vi "4-2 matrice NxM - matrice max - matrice 100x.vi"(0 "colonna\nsize":i32=4, 1 "riga\nsize":i32=3) -> (2 "Array moltiplicazione":dbl[](array[numeric]) format="%#_3g", 3 "Array massimi":dbl[](array[numeric]) format="%#_3g", 4 "Array":dbl[][](array[numeric]) format="%#.2g")   [LabVIEW 2012]
panel:
  out "Waveform Graph":cluster{dbl, dbl, dbl[][]}(graph)
  out "c(i)":dbl[](array[numeric]) format="%#_3g"
  out "b(i)":dbl[](array[numeric]) format="%#_3g"
  out "a(i)":dbl[](array[numeric]) format="%#_3g"
  # "Realizzare, mediante un generatore di numeri casuali,\n una matrice 3xN [a(i), b(i), c(i) con i che varia  da 0 a N-1] con N impostabile da pannello .\n\n Utilizzando la matrice generata dal SubVi precedente, generare due vettori\n  A(i) e B(i)  [0 <= i <= N-1] dove A(i) = Max [a(i),b(i),c(i)]  e B(i) = 100*[b(i) + c(N-1-i)]\n\nVisualizzare in un grafico i vettori a(i), b(i) e A(i)"
  # "DOMANDE: \n- nel ciclo for per la creazione di A(i), con l'indicizzazione abilitata in ingresso, \nil programma confronta automaticamente la prima, poi la seconda e infine la terza\nriga del vettore in ingresso, se invece collego l'indice di Array Subset all'indice del \nciclo, il confronto parte la prima volta dall'elemento 0-0, poi dall'elemento 1-1 e poi dal\n2-2 (che non c' quindi viene passato in uscita 0). Perch? Cosa devo cambiare perch \nfunzioni se l'indicizzazione non  abilitata?\n- nella creazione di B(i), ogni tanto la somma delle componenti non  esatta ( inferiore di 1 unit),\nperch? Il fatto che se rappresento le componenti di B(i) come decimali ottengo cifre sgnificative\ndopo la virgola  dovuto solo al fatto che i numeri random sono generati con molte cifre?"
  # "RISPOSTE:\n- per ottenere lo stesso risultato con l'indicizzazione non abilitata devo fare \"add dimension\" su \"array subset\",\ncollegare l'indice i del ciclo al primo indice di array subset e lasciare scollegato il secondo. Se faccio come nel\ntesto della domanda vengono confrontati gli elementi di uno stesso vettore.\n-  dovuto al fatto che i numeri random sono generati con molte cifre decimali, se la parte decimale supera 5\nil risultato viene arrotondato all'intero successivo."
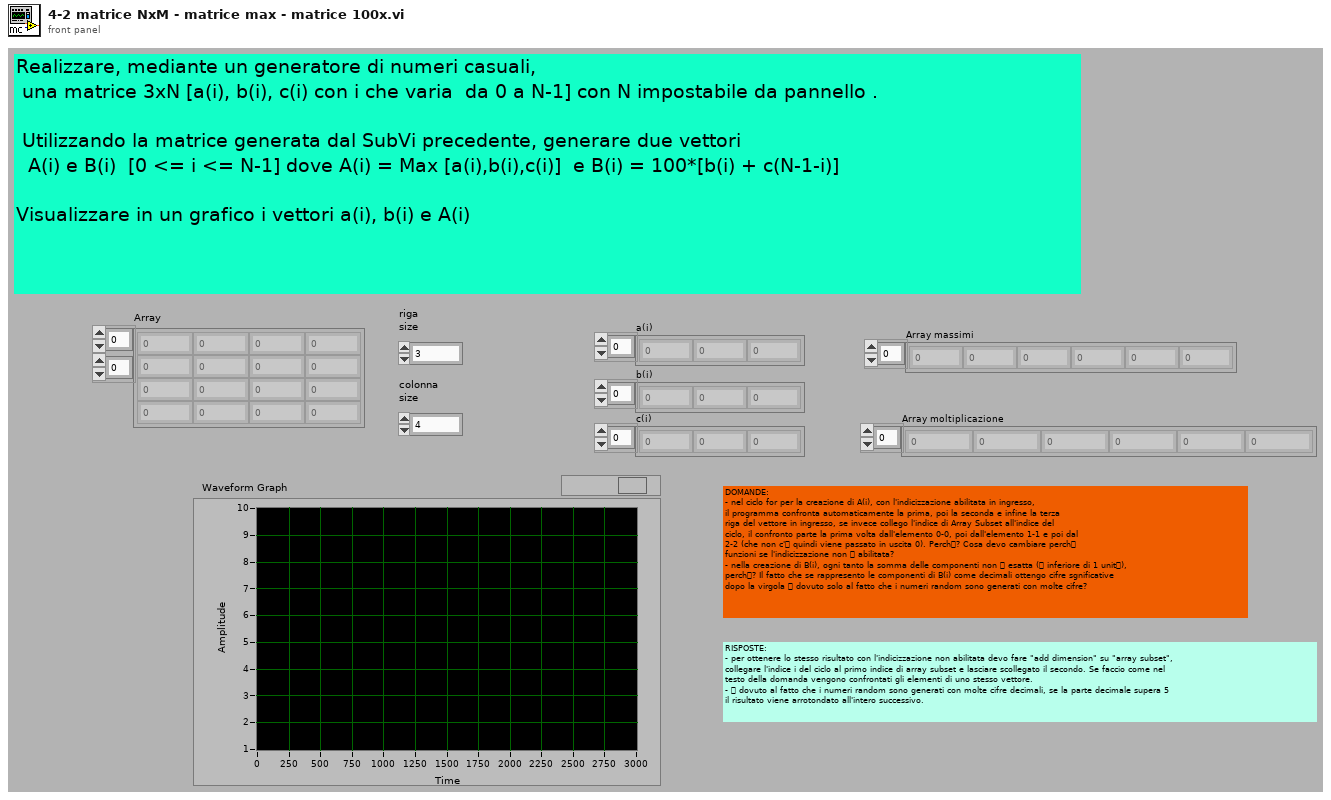
[diagram p1: front panel]
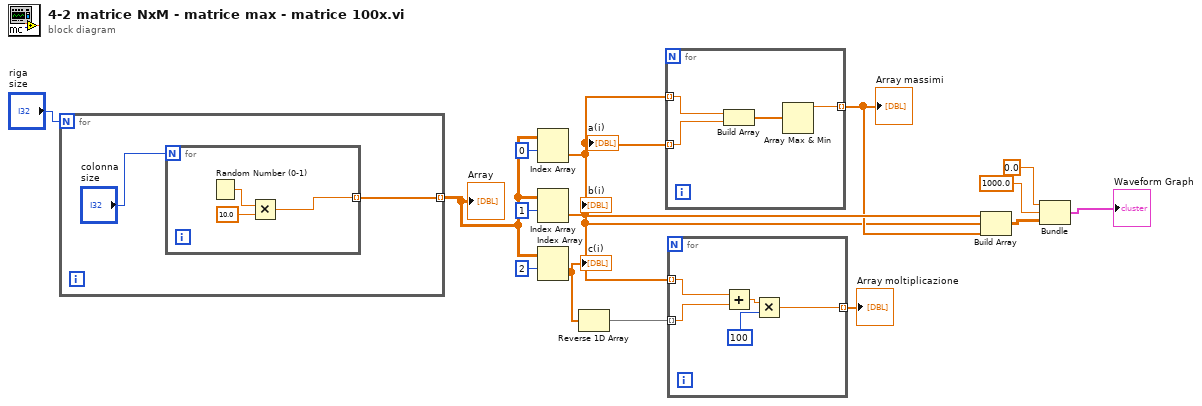
[diagram p0: block diagram]
diagram:
  n1 = for {
    N: "riga\nsize" -> [_]
    tunnel: [w16] -> w15 mode=indexing
    n2 = for {
      N: "colonna\nsize" -> [_]
      tunnel: [w20] -> w16 mode=indexing
      n3 = Random Number (0-1)() -> (number: 0 to 1=w19:dbl)
      n4 = Multiply(x=w19, y=10.0) -> (x*y=w20:dbl)
    }
  }
  "Array" <- w15
  n5 = Index Array(array=w15, index (row)=0) -> (element=w8:dbl[])  [unwired: 1 in]
  "a(i)" <- w8
  n6 = Index Array(array=w15, index (row)=1) -> (element=w6:dbl[])  [unwired: 1 in]
  "b(i)" <- w6
  n7 = Index Array(array=w15, index (row)=2) -> (element=w11:dbl[])  [unwired: 1 in]
  "c(i)" <- w11
  n8 = Reverse 1D Array(array=w11) -> (reversed array=w10:dbl[])
  n9 = for {
    tunnel: w8 -> [w24] mode=indexing
    tunnel: w6 -> [w23] mode=indexing
    tunnel: [w21] -> w7 mode=indexing
    n10 = Build Array(w24, w23) -> (w22:dbl[])
    n11 = Array Max & Min(array=w22) -> (max value=w21:dbl)  [unwired: 3 out]
  }
  "Array massimi" <- w7
  n12 = for {
    tunnel: w6 -> [w27] mode=indexing
    tunnel: w10 -> [w26] mode=indexing
    tunnel: [w25] -> w9 mode=indexing
    n13 = Add(x=w27, y=w26) -> (x+y=w29:dbl)
    n14 = Multiply(x=w29, y=100) -> (x*y=w25:dbl)
  }
  "Array moltiplicazione" <- w9
  n15 = Build Array(w8, w6, w7) -> (w5:dbl[][])
  n16 = Bundle(0.0, 1000.0, w5) -> (→"Waveform Graph":cluster{dbl, dbl, dbl[][]})  [unwired: 1 in]
